vi "run_chatcompletion.vi"(0 "chatcompletion_llm_interface in":refnum<class "llm_openai_chatmodels.lvclass">, 5 "Messages":refnum<class "abstract_message_base.lvclass">[](array[class]), 11 "error in (no error)":errorcluster) -> (4 "chatcompletion_llm_interface out":refnum<class "llm_openai_chatmodels.lvclass">, 6 "chat response":string, 15 "error out":errorcluster)   [LabVIEW 2020, in "llm_openai_chatmodels.lvclass"]
uses:
  llm_openai_chatmodels.lvclass
  abstract_message_base/abstract_message_base.lvclass
  <vilib>/httpClient/POSTBuffer.vi
  <vilib>/httpClient/LabVIEWHTTPClient.lvlib
panel:
  out "body":string
  out "headers":string
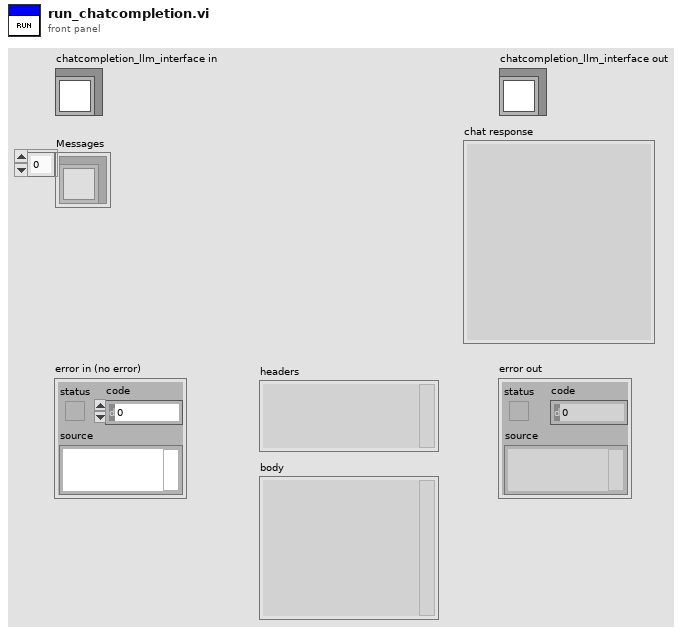
[diagram p1: front panel]
types:
  T1 = typedef "LabVIEWHTTPClient.lvlib/ClientHandle.ctl" = refnum<k1>
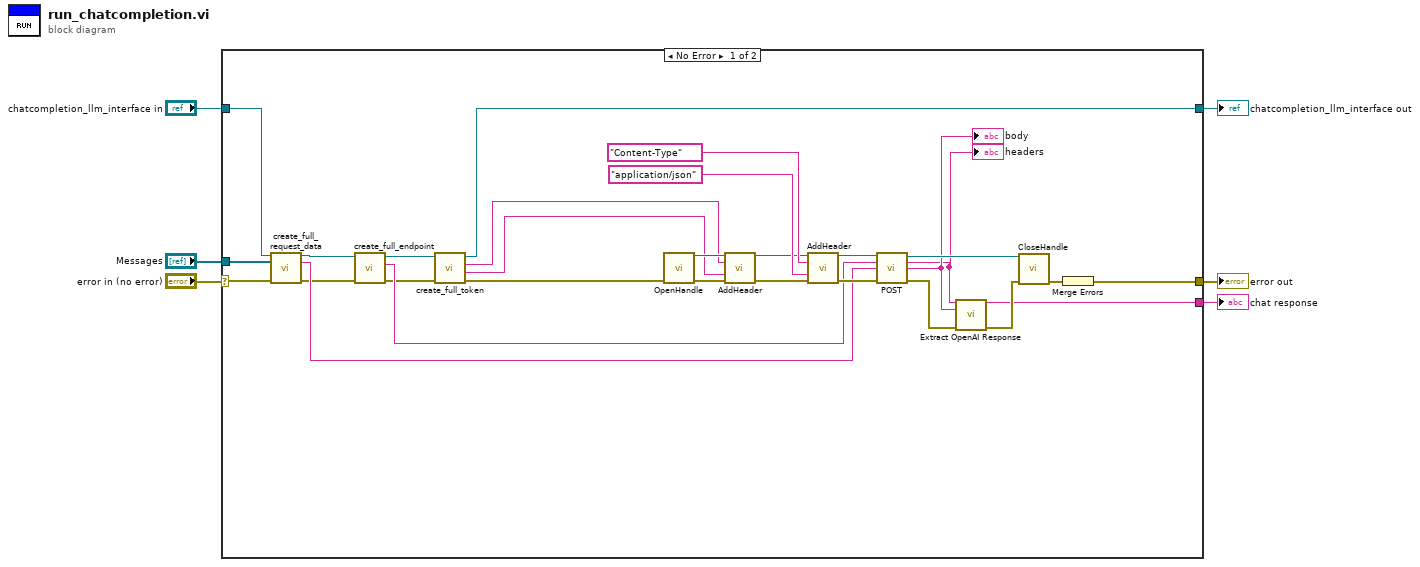
[diagram p0: block diagram]
diagram:
  n1 = case shown="No Error" "error in (no error)" {
    selector: "error in (no error)" -> [w17 w37]
    tunnel: [w20 w37] -> w5
    tunnel: "chatcompletion_llm_interface in" -> [w19 w36]
    tunnel: [w9 w36] -> w3
    tunnel: [w23 _] -> w2
    tunnel: "Messages" -> [w18 _]
    frame No Error {
      n2 = call-dynamic "create_full_request_data.vi"("llm_openai_chatmodels in"=w19, "Messages"=w18, "error in (no error)"=w17) -> ("llm_openai_chatmodels out"=w15:refnum<class "llm_openai_chatmodels.lvclass">, "Request Data"=w16:string, "error out"=w14:errorcluster)  [unwired: 10 in]
      n3 = call-dynamic "create_full_endpoint.vi"("error in (no error)"=w14, "llm_openai_chatmodels in"=w15) -> ("error out"=w12:errorcluster, "endpoint"=w13:string, "llm_openai_chatmodels out"=w10:refnum<class "llm_openai_chatmodels.lvclass">)  [unwired: 7 in]
      n4 = call-dynamic "create_full_token.vi"("error in (no error)"=w12, "llm_openai_chatmodels in"=w10) -> ("error out"=w11:errorcluster, "token"=w7:string, "header"=w8:string, "llm_openai_chatmodels out"=w9:refnum<class "llm_openai_chatmodels.lvclass">)  [unwired: 6 in]
      n5 = call <vilib>:"OpenHandle.vi"("error in (no error)"=w11) -> ("client handle out"=w35:T1, "error out"=w34:errorcluster)  [unwired: 13 in]
      n6 = call <vilib>:"AddHeader.vi"("client handle"=w35, "header"=w8, "value"=w7, "error in (no error)"=w34) -> ("client handle out"=w31:T1, "error out"=w29:errorcluster)  [unwired: 10 in]
      n7 = call <vilib>:"AddHeader.vi"("client handle"=w31, "header"="Content-Type", "value"="application/json", "error in (no error)"=w29) -> ("client handle out"=w30:T1, "error out"=w28:errorcluster)  [unwired: 10 in]
      n8 = call-poly <vilib>:"POST.vi"("client handle"=w30, "url"=w13, "buffer"=w16, "error in (no error)"=w28) -> ("client handle out"=w26:T1, "headers"=w21:string, "body"=w22:string, "error out"=w25:errorcluster)  [unwired: 8 in]
      "headers" <- w21
      "body" <- w22
      n9 = call "Extract OpenAI Response.vi"("headers"=w21, "body"=w22, "error in"=w25) -> ("value"=w23:string, "error out"=w24:errorcluster)  [unwired: 11 in]
      n10 = call <vilib>:"CloseHandle.vi"("client handle"=w26, "error in (no error)"=w24) -> ("error out"=w27:errorcluster)  [unwired: 13 in]
      n11 = Merge Errors(w27) -> (w20:errorcluster)
    }
    frame Error {
    }
  }
  "error out" <- w5
  "chatcompletion_llm_interface out" <- w3
  "chat response" <- w2
